vi "Initialize Synchronization Device.vi"(8 "error in (no error)":errorcluster, 11 "Application in":refnum<class "Application.lvclass">) -> (0 "error out":errorcluster, 3 "Application out":refnum<class "Application.lvclass">)   [LabVIEW 2015]
uses:
  User Interface/Splash Screen Messages/Update Status Msg/Update Status Msg.lvclass
  Hardware/Synchronization Device/Synchronization Device.lvclass
  <vilib>/ActorFramework/Actor/Actor.lvclass
  Application.lvclass
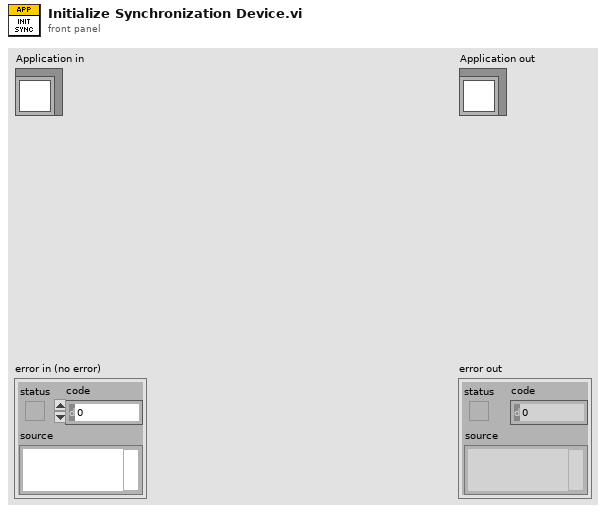
[diagram p1: front panel]
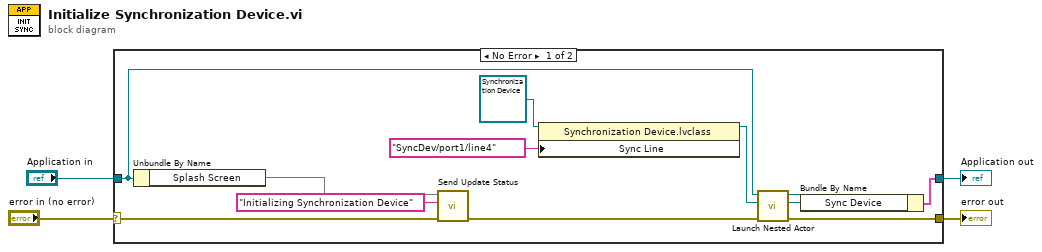
[diagram p0: block diagram]
diagram:
  n1 = case shown="No Error" "error in (no error)" {
    selector: "error in (no error)" -> [w11 w18]
    tunnel: [w10 w18] -> w3
    tunnel: [w12 w17] -> w1
    tunnel: "Application in" -> [w6 w17]
    frame No Error {
      n2 = Unbundle By Name(w6) -> ("Splash Screen"=w14)
      n3 = call "Send Update Status.vi"("error in (no error)"=w11, "Status Message"="Initializing Synchronization Device", "Message Enqueuer"=w14) -> ("error out"=w16:errorcluster)  [unwired: 7 in, 1 out]
      n4 = property class="Synchronization Device.lvclass"(reference=refnum<class "Synchronization Device.lvclass"> refnum ("Synchronization Device.lvlib:Synchronization Device.lvclass"), "Sync Line"=tag "SyncDev/port1/line4" ("lines")) -> (reference out=w7:refnum<class "Synchronization Device.lvclass">)  [unwired: 1 in, 1 out]
      n5 = call <vilib>:"Launch Nested Actor.vi"("error in (no error)"=w16, "Nested Actor"=w7, "Caller Actor in"=w6) -> ("error out"=w10:errorcluster, "Nested Actor's Enqueuer"=w13:refnum<class "Message Enqueuer.lvclass">, "Caller Actor out"=w5:refnum<class "Application.lvclass">)  [unwired: 6 in]
      n6 = Bundle By Name(cluster=w5, "Sync Device"=w13) -> (w12:cluster{})
    }
    frame Error {
    }
  }
  "error out" <- w3
  "Application out" <- w1
